vi "combine_two_u16.vi"(6 "Encode_1_w2":u16, 9 "Encode_1_w1":u16, 10 "forward":bool, 11 "little endian":bool) -> (2 "number":u32, 3 "Array":bool[](array[boolean]))   [LabVIEW 2019]
panel:
  out "Boolean array 2":bool[](array[boolean])
  out "Boolean array":bool[](array[boolean])
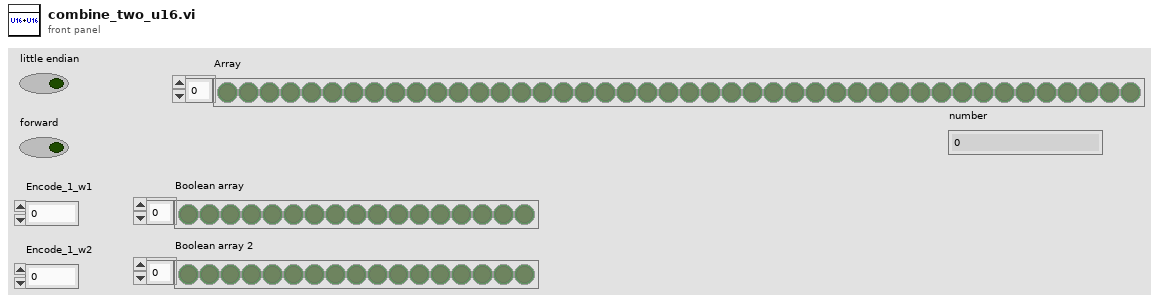
[diagram p1: front panel]
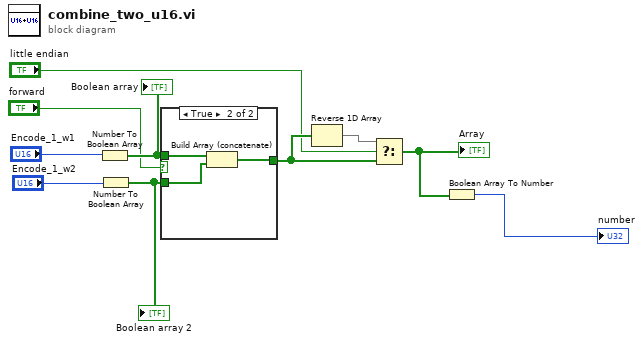
[diagram p0: block diagram]
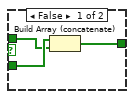
[diagram p2: hidden frame]
diagram:
  n1 = Number To Boolean Array(number="Encode_1_w1") -> (Boolean array=w6:bool[])
  "Boolean array" <- w6
  n2 = Number To Boolean Array(number="Encode_1_w2") -> (Boolean array=w7:bool[])
  "Boolean array 2" <- w7
  n3 = case shown="True" "forward" {
    tunnel: w6 -> [w12 w16]
    tunnel: w7 -> [w13 w15]
    tunnel: [w11 w14] -> w10
    frame False {
      n4 = Build Array (concatenate)(w13, w12) -> (w11:bool[])
    }
    frame True {
      n5 = Build Array (concatenate)(w16, w15) -> (w14:bool[])
    }
  }
  n6 = Reverse 1D Array(array=w10) -> (reversed array=w9:bool[])
  n7 = Select(t=w9, s="little endian", f=w10) -> (s? t:f=w2:bool[])
  "Array" <- w2
  n8 = Boolean Array To Number(Boolean array=w2) -> (number=→"number":u32)
